vi "Write motorData.vi"(8 "error in (no error)":errorcluster, 10 "motorData":T1={"Velo (RPM)"=0, "MotorTemp(C)"=0, "CtrlTemp(C)"=0, "DcLinkVolt(V)"=0.0, "ErrorCode"=0.0, "isAlive"=FALSE, "motorControllerState"=1, "motorStatus"={"isReady"=FALSE, "isOn"=FALSE, "isOperEn"=FALSE, "isFault"=FALSE, "isVoltEn"=FALSE, "targetReached"=FALSE, "isWarning"=FALSE}} {"motorControllerState" items=["unknown"=1, "boot-up"=0, "stopped"=4, "operational"=5, "pre-operational"=127, "connection lost"=128]}, 11 "MotorController in":refnum<class "MotorController.lvclass">) -> (0 "error out":errorcluster, 3 "MotorController out":refnum<class "MotorController.lvclass">)   [LabVIEW 2018, in "MotorController.lvclass"]
uses:
  MotorController.lvclass
  MotorData.ctl
  MotorStatus.ctl
  MotorController.lvclass/MotorController.ctl
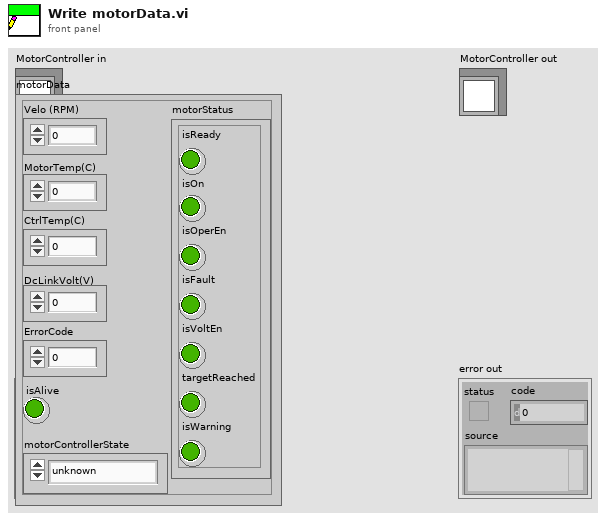
[diagram p1: front panel]
types:
  T1 = typedef "MotorData.ctl" = cluster{"Velo (RPM)":i32, "MotorTemp(C)":u8, "CtrlTemp(C)":u8, "DcLinkVolt(V)":dbl, "ErrorCode":dbl, "isAlive":bool, "motorControllerState":u16, "motorStatus":T2}
  T2 = typedef "MotorStatus.ctl" = cluster{"isReady":bool, "isOn":bool, "isOperEn":bool, "isFault":bool, "isVoltEn":bool, "targetReached":bool, "isWarning":bool}
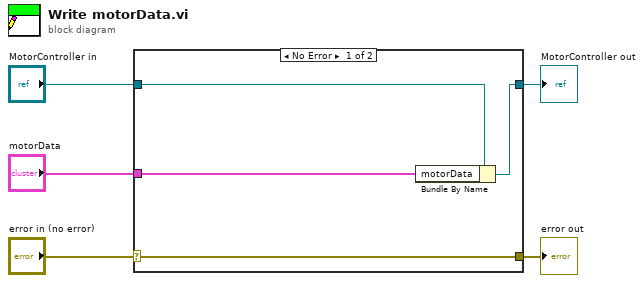
[diagram p0: block diagram]
diagram:
  n1 = case shown="No Error" "error in (no error)" {
    selector: "error in (no error)" -> [w9 w10]
    tunnel: [w9 w10] -> w4
    tunnel: [w7 w11] -> w2
    tunnel: "MotorController in" -> [w8 w11]
    tunnel: "motorData" -> [w6 _]
    frame No Error {
      n2 = Bundle By Name(cluster=w8, "motorData"=w6) -> (w7:refnum<class "MotorController.lvclass">)
    }
    frame Error {
    }
  }
  "error out" <- w4
  "MotorController out" <- w2
